vi "Configure Measurement (Reflection Measurement - DTF).vi"(0 "VISA resource name":refnum<visa-resource-name>, 1 "Distance Unit (0: Meter)":i32(ring) items=["Meter", "Feet"], 5 "Distance Start (0.12 meters)":dbl=0.12, 9 "Distance Stop (0.15 meter)":dbl=0.15, 11 "error in (no error)":errorcluster) -> (4 "VISA resource name out":refnum<visa-resource-name>, 15 "error out":errorcluster)   [LabVIEW 2022 SP3, in "Agilent N934X Series.lvlib"]
doc: "Configures the Distance to Fault Measurement setting of Reflection Measurement Option.\n\nNote:\nThis VI is only applicable for N9321C, N9322C, N9323C, N9324C models"
uses:
  <instrlib>/Agilent N934X Series/Agilent N934X Series.lvlib
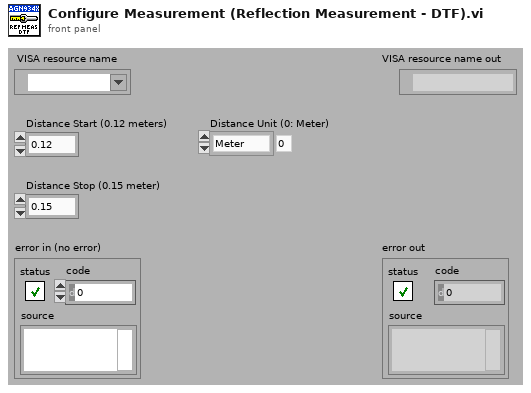
[diagram p1: front panel]
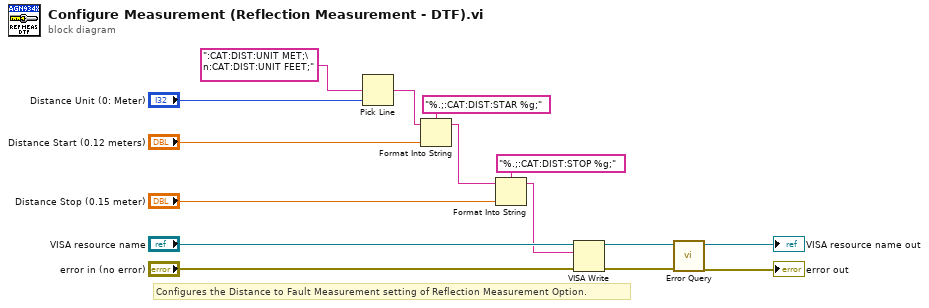
[diagram p0: block diagram]
diagram:
  # "Configures the Distance to Fault Measurement setting of Reflection Measurement Option."
  n1 = Pick Line(multi-line string=":CAT:DIST:UNIT MET;\n:CAT:DIST:UNIT FEET;", line index="Distance Unit (0: Meter)") -> (output string=w2:string)  [unwired: 1 in]
  n2 = Format Into String(format string="%.;:CAT:DIST:STAR %g;", initial string=w2, "Distance Start (0.12 meters)") -> (resulting string=w13:string)  [unwired: 1 in, 1 out]
  n3 = Format Into String(format string="%.;:CAT:DIST:STOP %g;", initial string=w13, "Distance Stop (0.15 meter)") -> (resulting string=w1:string)  [unwired: 1 in, 1 out]
  n4 = VISA Write(VISA resource name="VISA resource name", write buffer=w1, error in (no error)="error in (no error)") -> (VISA resource name out=w6:refnum<visa-resource-name>, error out=w5:errorcluster)  [unwired: 1 out]
  n5 = call <instrlib>:"Error Query.vi"("error in (no error)"=w5, "VISA resource name"=w6) -> ("error out"=→"error out":errorcluster, "VISA resource name out"=→"VISA resource name out":refnum<visa-resource-name>)  [unwired: 6 in, 2 out]
